vi "Modules Config.vi"(10 "Name":string, 11 "Module In":T1={"Names"={"Module Name"="", "Set Value"="", "Real Value"="", "FB Value"="", "Unit"="", "Identifier"="", "IdentifierW"="", "Decimal"="位数", "AS"=FALSE, "AR"=FALSE, "Con"=FALSE}, "Data"=[], "Digit"=0.0}) -> (2 "OK？":bool, 3 "Module Out":T1={"Names"={"Module Name"="", "Set Value"="", "Real Value"="", "FB Value"="", "Unit"="", "Identifier"="", "IdentifierW"="", "Decimal"="位数", "AS"=FALSE, "AR"=FALSE, "Con"=FALSE}, "Data"=[], "Digit"=0.0})   [LabVIEW 2020]
uses:
  0007 Controls/Data Modules.ctl
  0007 Controls/Data Element Single.ctl
  Global/Data Global/SDQ Data Type.ctl
panel:
  in  "InputBox":dbl
  in  "OK":bool
  in  "Cancel":bool
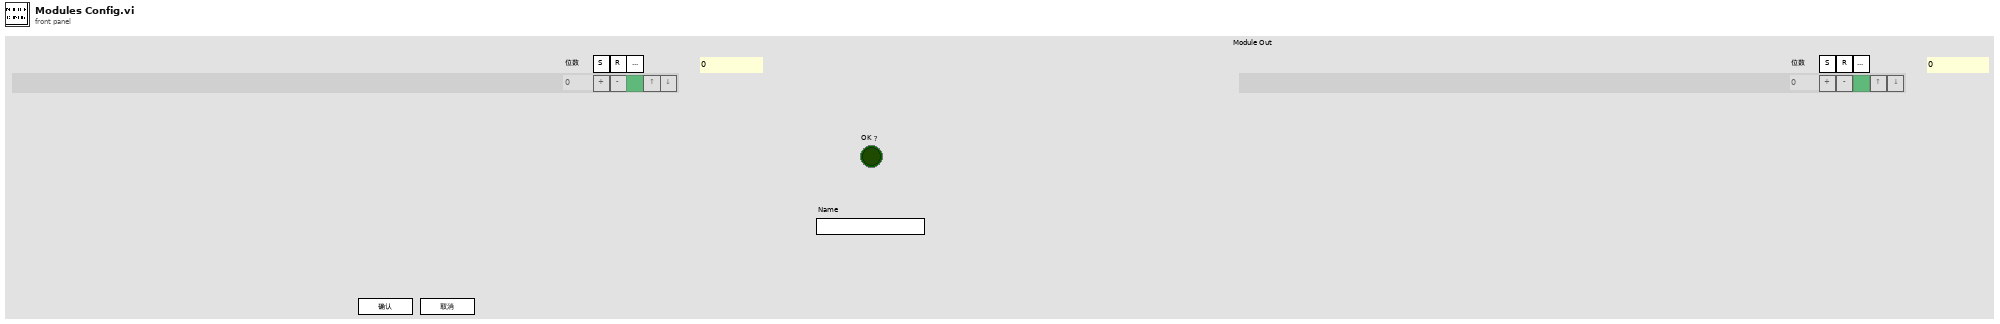
[diagram p1: front panel]
types:
  T1 = typedef "Data Modules.ctl" = cluster{"Names":cluster{"Module Name":string, "Set Value":string, "Real Value":string, "FB Value":string, "Unit":string, "Identifier":string, "IdentifierW":string, "Decimal":string, "AS":bool, "AR":bool, "Con":bool}, "Data":T2[], "Digit":dbl}
  T2 = typedef "Data Element Single.ctl" = cluster{"Name":string, "Set Value":string, "Real Value":string, "FB Value":string, "Unit":string, "Identifier":string, "Write Name":string, "Decimal":u16, "AS":bool, "AR":bool, "ALM":bool, "Up":bool, "Down":bool}
  T3 = typedef "SDQ Data Type.ctl" = cluster{"CAN Length":string, "CAN Name":string, "CAN ID":string, "CAN Type":string, "Test Item":string, "Byte Order":string, "Instruction":string, "Control Type":string, "Group":string, "Offset":dbl, "Coefficient":dbl, "Write Enable":bool, "Lable Type":string, "Key?":string, "Set Value":string, "Upper":dbl, "Lower":dbl, "Unit":string, "Formula":string, "Test Item Type":string, "Length":i32, "Address":string, "Name":string, "Identifier":string, "Data Type":string, "Enumerate?":string, "Enumerate List":string, "Data":string, "Source":string}
  T4 = cluster{"Active Row":i32, "Module In":T1, "TimeOut":i32, "List Visible":bool, "OK?":bool, "Active Column":i32, "Receive Data":map{string, T3}, "Data":refnum<vi>, "Name":string}
  T5 = enum8{"Enabled", "Disabled", "Disabled and Grayed Out"}
  T6 = enum32{"Invalid", "Default", "Floating", "Floating/Auto-Hide", "Modal"}
  T7 = cluster{"Name":bool, "Set Value":bool, "Real Value":bool, "FB Value":bool, "Unit":bool, "Identifier":bool, "Write Name":bool, "Decimal":bool, "AS":bool, "AR":bool, "ALM":bool, "Up":bool, "Down":bool}[]
  T8 = typedef "LVPoint32TypeDef.ctl" = cluster{"Horizontal":i32, "Vertical":i32}
  T9 = typedef "LVPositionTypeDef.ctl" = cluster{"Left":i32, "Top":i32}
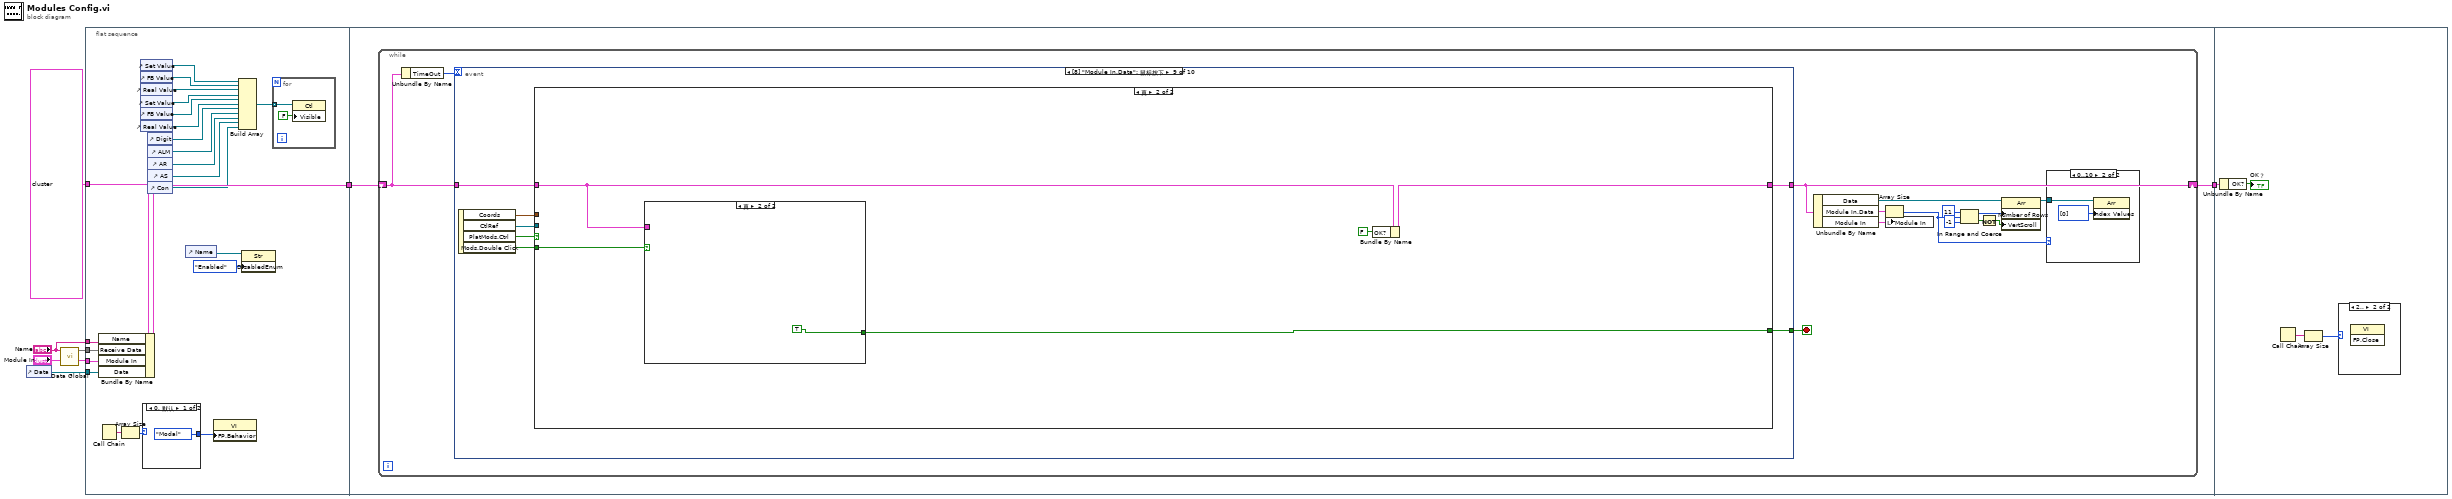
[diagram p0: block diagram]
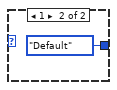
[diagram p2: hidden frame]
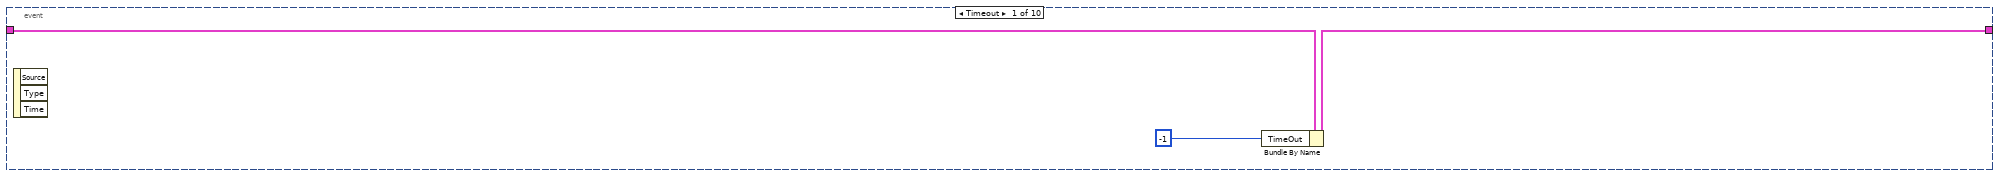
[diagram p3: hidden frame]
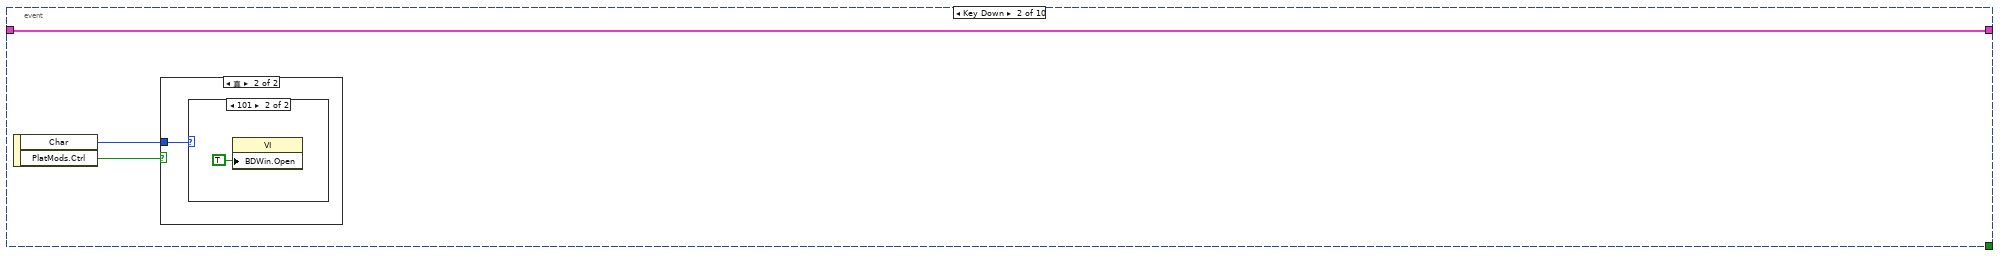
[diagram p4: hidden frame]
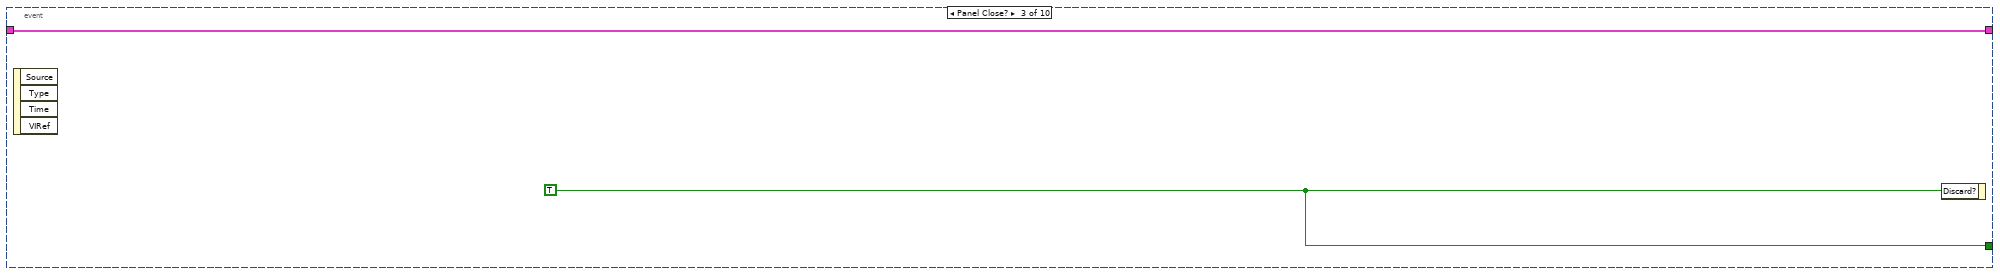
[diagram p7: hidden frame]
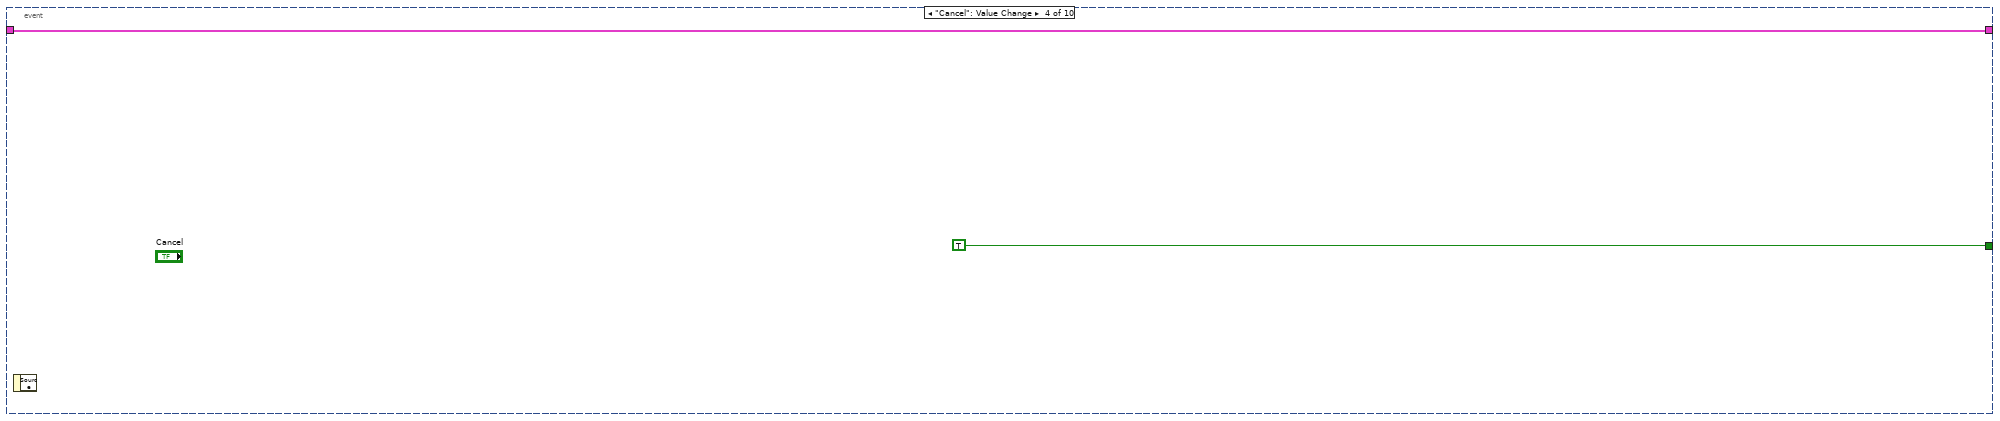
[diagram p8: hidden frame]
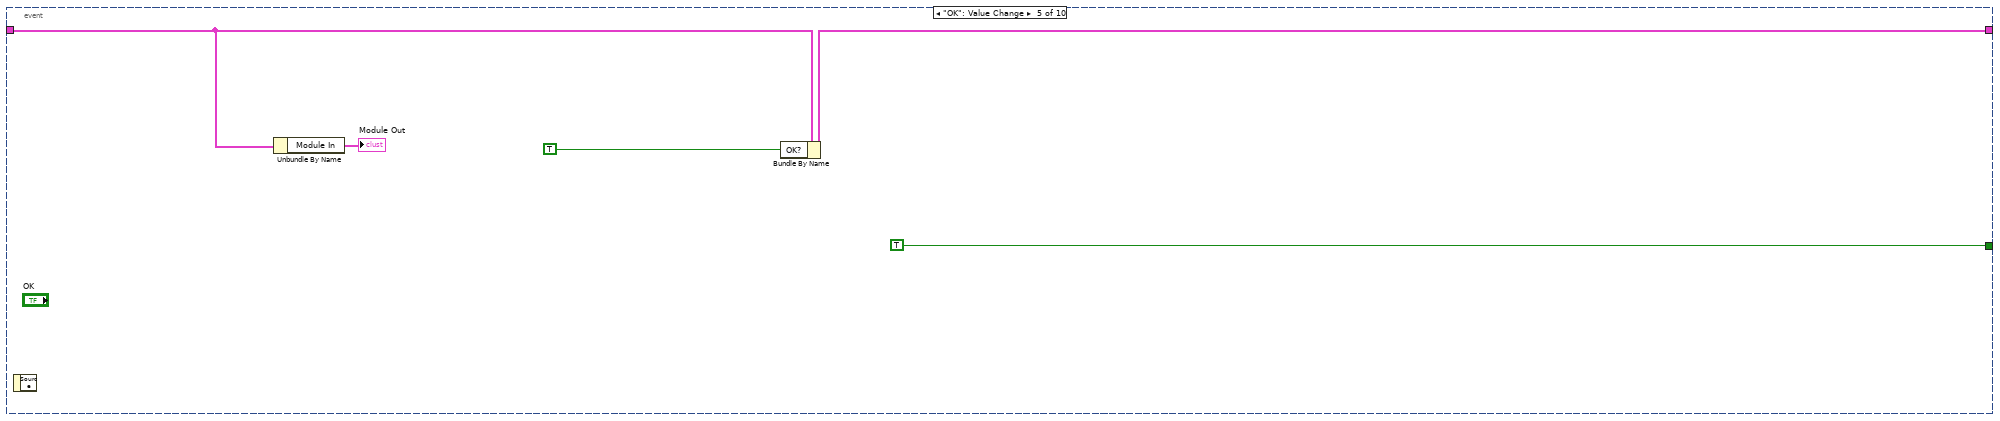
[diagram p9: hidden frame]
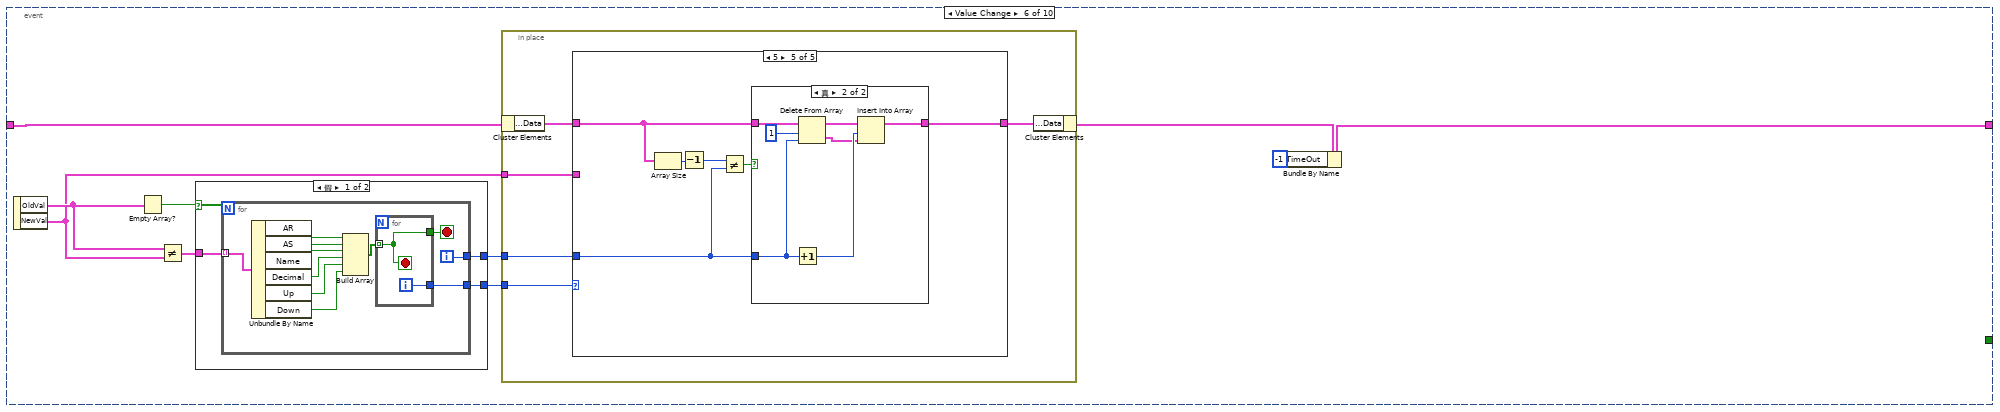
[diagram p10: hidden frame]
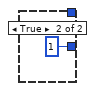
[diagram p11: hidden frame]
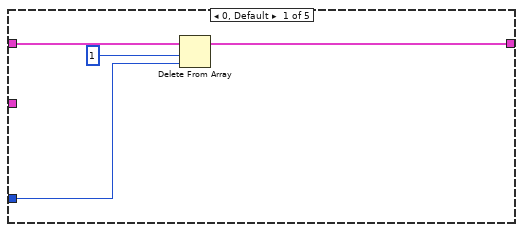
[diagram p12: hidden frame]
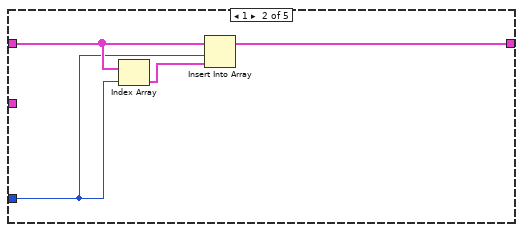
[diagram p13: hidden frame]
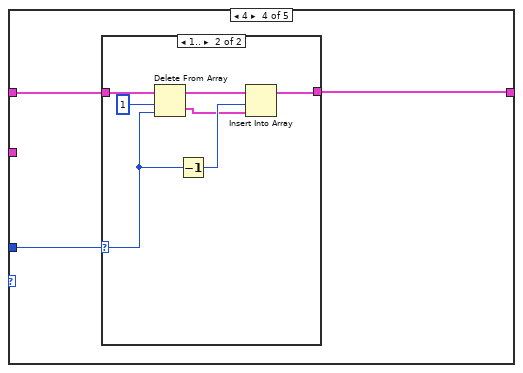
[diagram p15: hidden frame]
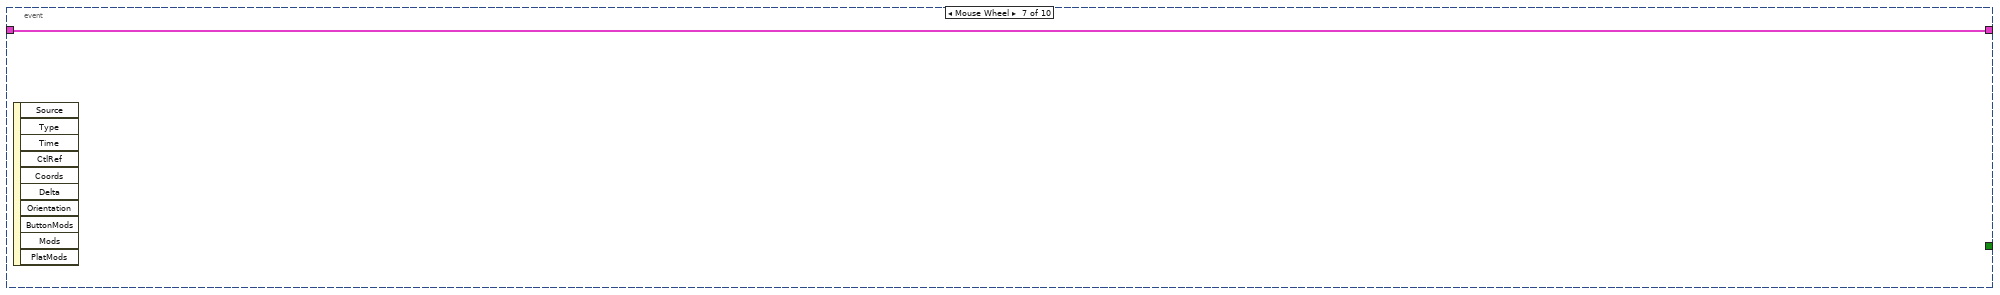
[diagram p18: hidden frame]
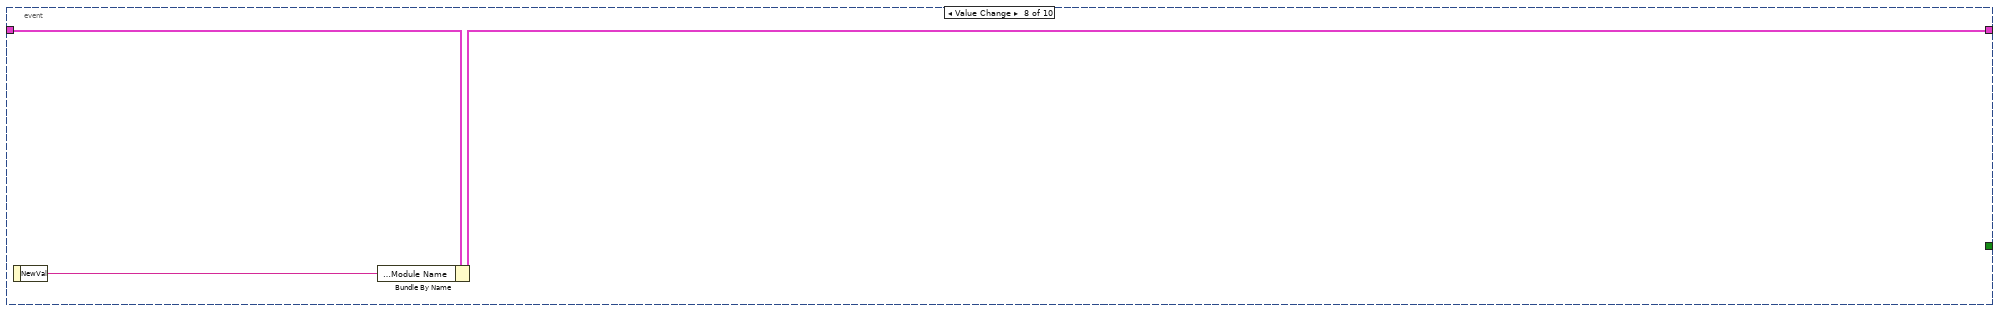
[diagram p19: hidden frame]
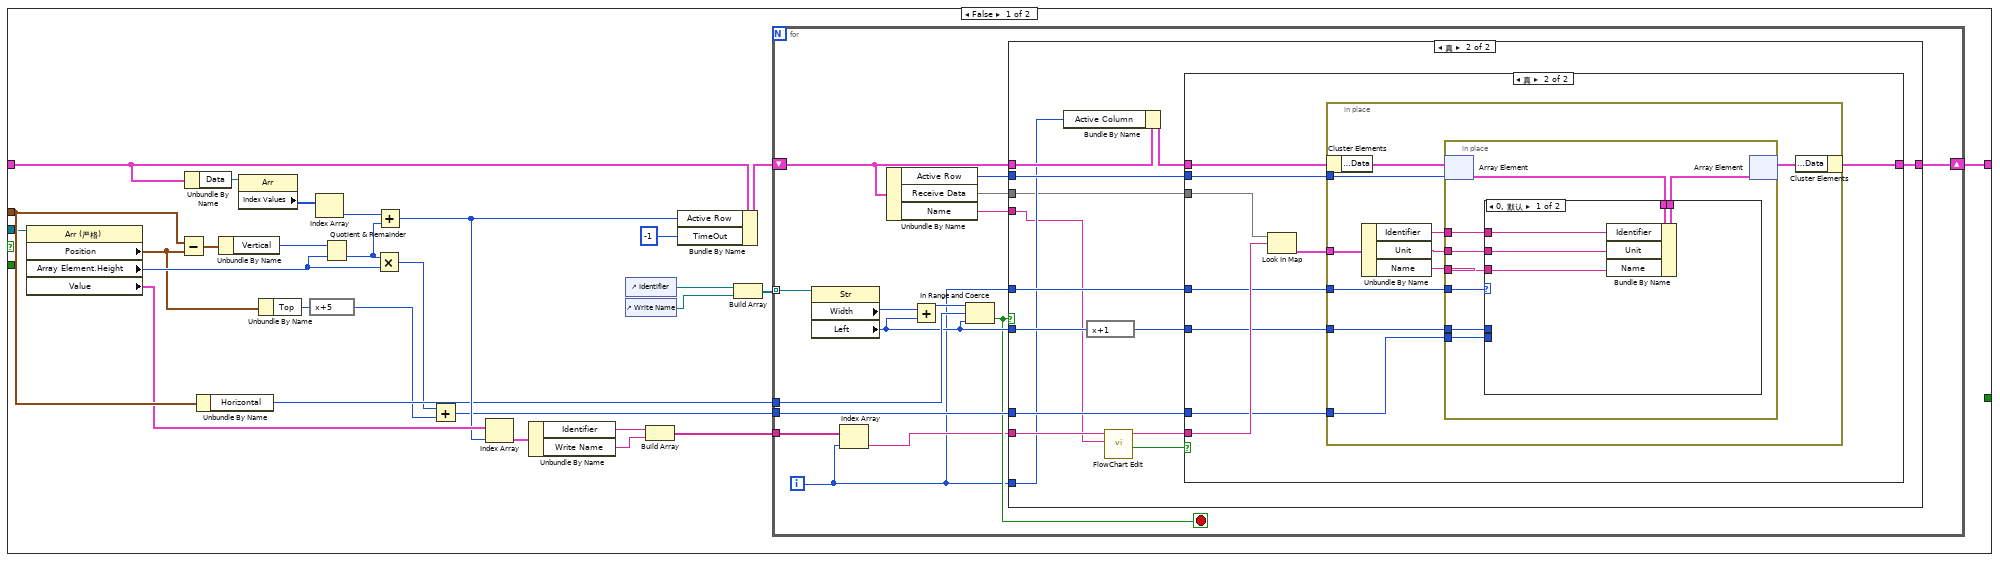
[diagram p20: hidden frame]
diagram:
  n1 = control-ref of="Data"() -> (w3:refnum<vi>)
  n2 = call "Data Global.vi"("Name"="Name") -> ("Data Out"=w2:map{string, T3})  [unwired: 7 in, 3 out]
  n3 = flat-sequence {
    tunnel: "Module In" -> [w28]
    tunnel: T4 {"Active Row"=0, "Module In"={"Names"={"Module Name"="", "Set Value"="", "Real Value"="", "FB Value"="", "Unit"="", "Identifier"="", "IdentifierW"="", "Decimal"="位数", "AS"=FALSE, "AR"=FALSE, "Con"=FALSE}, "Data"=[], "Digit"=0.0}, "TimeOut"=50, "List Visible"=FALSE, "OK?"=FALSE, "Active Column"=50, "Receive Data"={}, "Data"=refnum, "Name"=""} -> [w30]
    tunnel: [w29] -> w5
    tunnel: w2 -> [w25]
    tunnel: w3 -> [w24]
    tunnel: "Name" -> [w14]
    tunnel: w5 -> [w36]
    tunnel: [w35] -> w4
    tunnel: w4 -> [w266]
    frame #0 {
      n4 = Bundle By Name(cluster=w30, "Name"=w14, "Receive Data"=w25, "Module In"=w28, "Data"=w24) -> (w29:T4)
      n5 = Call Chain() -> (call chain=w27:string[])
      n6 = Array Size(array=w27) -> (size(s)=w26:i32)
      n7 = control-ref of="Set Value"() -> (w16:refnum<vi>)
      n8 = control-ref of="FB Value"() -> (w17:refnum<vi>)
      n9 = control-ref of="Real Value"() -> (w18:refnum<vi>)
      n10 = control-ref of="Set Value"() -> (w19:refnum<vi>)
      n11 = control-ref of="FB Value"() -> (w20:refnum<vi>)
      n12 = control-ref of="Real Value"() -> (w21:refnum<vi>)
      n13 = case shown="0, 默认" w26 {
        tunnel: [T6."Modal" ("前面板窗口:动作") T6."Default" ("前面板窗口:动作")] -> w15
        frame 0, Default {
        }
        frame 1 {
        }
      }
      n14 = control-ref of="AR"() -> (w12:refnum<vi>)
      n15 = control-ref of="Con"() -> (w10:refnum<vi>)
      n16 = control-ref of="Digit"() -> (w22:refnum<vi>)
      n17 = control-ref of="ALM"() -> (w13:refnum<vi>)
      n18 = control-ref of="AS"() -> (w11:refnum<vi>)
      n19 = control-ref of="Name"() -> (w9:refnum<vi>)
      n20 = property class="VI"("FP.Behavior"=w15) -> ()  [unwired: 2 in, 2 out]
      n21 = Build Array(w16, w17, w18, w19, w20, w21, w22, w13, w12, w11, w10) -> (w23:refnum<vi>[])
      n22 = property class="Str"(reference=w9, "DisabledEnum"=T5."Enabled" ("禁用")) -> ()  [unwired: 1 in, 2 out]
      n23 = for {
        tunnel: w23 -> [w32] mode=indexing
        n24 = property class="Ctl"(reference=w32, "Visible"=FALSE ("可见")) -> ()  [unwired: 1 in, 2 out]
      }
    }
    frame #1 {
      n25 = while {
        shift-right: [w49] -> w35
        shift-left: w36 -> [w48]
        stop <- w50 stop-if-true
        n26 = Unbundle By Name(w48) -> ("TimeOut"=w47:i32)
        n27 = event shown="[8] \"Module In.Data\": 鼠标按下" {
          selector: _ -> [_ _ _ _ _ _ _ _ _ _]
          dyn-events: _ -> [_ _ _ _ _ _ _ _ _ _]
          timeout: w47 -> [_ _ _ _ _ _ _ _ _ _]
          tunnel: [_ _ w60 TRUE ("放弃？") TRUE ("放弃？") _ _ _ w138 _] -> w50
          tunnel: w48 -> [w53 w56 w59 w61 w66 w74 w134 w137 w141 w248]
          tunnel: [w52 w56 w59 w61 w64 w76 w134 w136 w142 w249] -> w49
          event Timeout {
            n28 = event-data() -> ()  [unwired: 1 in, 3 out]
            n29 = Bundle By Name(cluster=w53, "TimeOut"=-1) -> (w52:T4)
          }
          event Key Down {
            n30 = event-data() -> ("Char"=w55:i16, "PlatMods.Ctrl"=w54:bool)  [unwired: 1 in]
            n31 = case shown="真" w54 {
              tunnel: w55 -> [_ w57]
              frame False {
              }
              frame True {
                n32 = case shown="101" w57 {
                  frame 0, Default {
                  }
                  frame 101 {
                    n33 = property class="VI"("BDWin.Open"=TRUE ("程序框图窗口:打开")) -> ()  [unwired: 2 in, 2 out]
                  }
                }
              }
            }
          }
          event Panel Close? {
            w60 = TRUE ("放弃？")
            n34 = event-data() -> ()  [unwired: 1 in, 4 out]
            n35 = event-data("Discard?"=w60) -> ()  [unwired: 1 in, 1 out]
          }
          event "Cancel": Value Change {
            n36 = event-data() -> ()  [unwired: 1 in, 1 out]
          }
          event "OK": Value Change {
            n37 = event-data() -> ()  [unwired: 1 in, 1 out]
            n38 = Unbundle By Name(w66) -> ("Module In"=→"Module Out":T1)
            n39 = Bundle By Name(cluster=w66, "OK?"=TRUE) -> (w64:T4)
          }
          event Value Change {
            n40 = event-data() -> ("OldVal"=w73:T2[], "NewVal"=w71:T2[])  [unwired: 1 in]
            n41 = Empty Array?(array=w73) -> (empty?=w70:bool)
            n42 = Not Equal?(x=w73, y=w71) -> (x != y?=w72:T7)
            n43 = case shown="假" w70 {
              tunnel: [w80 _] -> w69
              tunnel: w72 -> [w79 _]
              tunnel: [w78 1] -> w68
              frame False {
                n44 = for {
                  tunnel: [w91] -> w80
                  tunnel: w79 -> [w90] mode=indexing
                  tunnel: [w84] -> w78
                  i -> [w91]
                  stop <- w85 stop-if-true
                  n45 = Unbundle By Name(w90) -> ("AR"=w89:bool, "AS"=w88:bool, "Name"=w87:bool, "Decimal"=w83:bool, "Up"=w82:bool, "Down"=w81:bool)
                  n46 = Build Array(w89, w88, w87, w83, w82, w81) -> (w86:bool[])
                  n47 = for {
                    tunnel: w86 -> [w93] mode=indexing
                    tunnel: [w93] -> w85
                    tunnel: [w92] -> w84
                    i -> [w92]
                    stop <- w93 stop-if-true
                  }
                }
              }
              frame True {
              }
            }
            n48 = in-place {
              in-place-border: w69 -> [w97]
              in-place-border: w68 -> [w96]
              in-place-border: w71 -> [w95]
              n49 = in-place-cluster #1(w74) -> ("Module In.Data"=w99:T2[])
              n50 = case shown="5" w96 {
                tunnel: w99 -> [w103 w106 _ w110 w122]
                tunnel: [w102 w107 w108 w109 w121] -> w98
                tunnel: w97 -> [w101 w104 _ w111 w120]
                tunnel: w95 -> [_ _ w108 _ _]
                frame 0, Default {
                  n51 = Delete From Array(array=w103, length=1 ("长度"), index=w101) -> (array with subset deleted=w102:T2[])  [unwired: 1 out]
                }
                frame 1 {
                  n52 = Index Array(array=w106, index=w104) -> (element=w105:T2)
                  n53 = Insert Into Array(array=w106, index=w104, new element=w105) -> (w107:T2[])
                }
                frame 2, 3 {
                }
                frame 4 {
                  n54 = case shown="1.." w111 {
                    selector: w111 -> [_ w114]
                    tunnel: [w112 w116] -> w109
                    tunnel: w110 -> [w112 w119]
                    frame 0, Default {
                    }
                    frame 1.. {
                      n55 = Delete From Array(array=w119, length=1 ("长度"), index=w114) -> (deleted portion=w115:T2[], array with subset deleted=w118:T2[])
                      n56 = Decrement(x=w114) -> (x-1=w117:i32)
                      n57 = Insert Into Array(array=w118, index=w117, new element=w115) -> (w116:T2[])
                    }
                  }
                }
                frame 5 {
                  n58 = Array Size(array=w122) -> (size(s)=w125:i32)
                  n59 = Decrement(x=w125) -> (x-1=w124:i32)
                  n60 = Not Equal?(x=w124, y=w120) -> (x != y?=w123:bool)
                  n61 = case shown="真" w123 {
                    tunnel: w122 -> [w126 w133]
                    tunnel: [w126 w127] -> w121
                    tunnel: w120 -> [_ w130]
                    frame False {
                    }
                    frame True {
                      n62 = Increment(x=w130) -> (x+1=w129:i32)
                      n63 = Delete From Array(array=w133, length=1 ("长度"), index=w130) -> (deleted portion=w128:T2[], array with subset deleted=w132:T2[])
                      n64 = Insert Into Array(array=w132, index=w129, new element=w128) -> (w127:T2[])
                    }
                  }
                }
              }
              n65 = in-place-cluster #1("Module In.Data"=w98) -> (w77:T4)
            }
            n66 = Bundle By Name(cluster=w77, "TimeOut"=-1) -> (w76:T4)
          }
          event Mouse Wheel {
            n67 = event-data() -> ()  [unwired: 1 in, 10 out]
          }
          event Value Change {
            n68 = event-data() -> ("NewVal"=w135:string)  [unwired: 1 in]
            n69 = Bundle By Name(cluster=w137, "Module In.Names.Module Name"=w135) -> (w136:T4)
          }
          event Mouse Down {
            n70 = event-data() -> ("Coords"=w144:T8, "CtlRef"=w143:refnum<vi>, "PlatMods.Ctrl"=w140:bool, "Mods.Double Click"=w139:bool)  [unwired: 1 in]
            n71 = case shown="真" w140 {
              tunnel: w144 -> [w172 _]
              tunnel: w143 -> [w171 _]
              tunnel: [w170 w241] -> w142
              tunnel: w141 -> [w148 w239]
              tunnel: w139 -> [_ w243]
              tunnel: [_ w242] -> w138
              frame False {
                n72 = property class="Arr (严格)"(reference=w171) -> ("Position"=w150:T9, "Array Element.Height"=w154:u32, "Value"=w163:T2[])  [unwired: 1 in, 2 out]
                n73 = Subtract(x=w172, y=w150) -> (x-y=w169:T8)
                n74 = Unbundle By Name(w148) -> ("Data"=w147:refnum<vi>)
                n75 = Unbundle By Name(w172) -> ("Horizontal"=w156:i32)
                n76 = Unbundle By Name(w169) -> ("Vertical"=w168:i32)
                n77 = property on="属性节点" class="Arr"(reference=w147) -> ("Index Values"=w165:u32[])  [unwired: 1 in, 2 out]
                n78 = Unbundle By Name(w150) -> ("Top"=w152:i32)
                n79 = expression code="x+5"(w152) -> (w149:i32)
                n80 = Index Array(array=w165) -> (element=w164:u32)  [unwired: 1 in]
                n81 = Quotient & Remainder(x=w168, y=w154) -> (floor(x/y)=w155:u32)  [unwired: 1 out]
                n82 = Multiply(x=w155, y=w154) -> (x*y=w153:u32)
                n83 = Add(x=w164, y=w155) -> (x+y=w162:u32)
                n84 = Add(x=w153, y=w149) -> (x+y=w151:u32)
                n85 = Index Array(array=w163, index=w162) -> (element=w167:T2)
                n86 = Unbundle By Name(w167) -> ("Identifier"=w161:string, "Write Name"=w160:string)
                n87 = control-ref of="Identifier"() -> (w146:refnum<vi>)
                n88 = control-ref of="Write Name"() -> (w145:refnum<vi>)
                n89 = Build Array(w161, w160) -> (w159:string[])
                n90 = Bundle By Name(cluster=w148, "Active Row"=w162, "TimeOut"=-1) -> (w157:T4)
                n91 = Build Array(w146, w145) -> (w158:refnum<vi>[])
                n92 = for {
                  tunnel: w159 -> [w176]
                  tunnel: w158 -> [w185] mode=indexing
                  tunnel: w156 -> [w184]
                  shift-right: [w183] -> w170
                  shift-left: w157 -> [w182]
                  tunnel: w151 -> [w178]
                  i -> [w174]
                  stop <- w177 stop-if-true
                  n93 = property class="Str"(reference=w185) -> ("Width"=w187:u32, "Left"=w179:i32)  [unwired: 1 in, 2 out]
                  n94 = Index Array(array=w176, index=w174) -> (element=w175:string)
                  n95 = Unbundle By Name(w182) -> ("Active Row"=w180:i32, "Receive Data"=w181:map{string, T3}, "Name"=w173:string)
                  n96 = Add(x=w187, y=w179) -> (x+y=w186:u32)
                  n97 = In Range and Coerce(upper limit=w186, x=w184, lower limit=w179) -> (In Range?=w177:bool)  [unwired: 1 out]
                  n98 = case shown="真" w177 {
                    tunnel: w175 -> [_ w202]
                    tunnel: w182 -> [w188 w201]
                    tunnel: [w188 w200] -> w183
                    tunnel: w181 -> [_ w190]
                    tunnel: w180 -> [_ w197]
                    tunnel: w174 -> [_ w196]
                    tunnel: w179 -> [_ w195]
                    tunnel: w178 -> [_ w194]
                    tunnel: w174 -> [_ w191]
                    tunnel: w173 -> [_ w189]
                    frame False {
                    }
                    frame True {
                      n99 = Bundle By Name(cluster=w201, "Active Column"=w191) -> (w192:T4)
                      n100 = expression code="x+1"(w195) -> (w193:i32)
                      n101 = call "FlowChart Edit.vi"("Name"=w189, "Identifier In"=w202) -> ("OK？"=w199:bool, "Identifier Out"=w198:string)  [unwired: 6 in, 2 out]
                      n102 = case shown="真" w199 {
                        tunnel: w192 -> [w203 w212]
                        tunnel: [w203 w211] -> w200
                        tunnel: w198 -> [_ w209]
                        tunnel: w190 -> [_ w210]
                        tunnel: w197 -> [_ w208]
                        tunnel: w196 -> [_ w206]
                        tunnel: w193 -> [_ w205]
                        tunnel: w194 -> [_ w204]
                        frame False {
                        }
                        frame True {
                          n103 = Look In Map(map=w210, key=w209) -> (value=w207:T3)  [unwired: 1 in, 1 out]
                          n104 = in-place {
                            in-place-border: w208 -> [w220]
                            in-place-border: w207 -> [w219]
                            in-place-border: w206 -> [w215]
                            in-place-border: w205 -> [w214]
                            in-place-border: w204 -> [w213]
                            n105 = in-place-cluster #2(w212) -> ("Module In.Data"=w222:T2[])
                            n106 = Unbundle By Name(w219) -> ("Identifier"=w218:string, "Unit"=w217:string, "Name"=w216:string)
                            n107 = in-place {
                              in-place-border: w218 -> [w228]
                              in-place-border: w217 -> [w227]
                              in-place-border: w216 -> [w226]
                              in-place-border: w215 -> [w225]
                              in-place-border: w214 -> [w224]
                              in-place-border: w213 -> [w223]
                              n108 = in-place-array #3(w222, w220) -> (w230:T2)
                              n109 = case shown="0, 默认" w225 {
                                tunnel: w230 -> [w235 w238]
                                tunnel: [w234 w237] -> w229
                                tunnel: w228 -> [w233 w236]
                                tunnel: w227 -> [w232 _]
                                tunnel: w226 -> [w231 _]
                                tunnel: w224 -> [_ _]
                                tunnel: w223 -> [_ _]
                                frame 0, Default {
                                n110 = Bundle By Name(cluster=w235, "Identifier"=w233, "Unit"=w232, "Name"=w231) -> (w234:T2)
                                }
                                frame 1 {
                                n111 = Bundle By Name(cluster=w238, "Write Name"=w236) -> (w237:T2)
                                }
                              }
                              n112 = in-place-array #3(w229) -> (w221:T2[])  [unwired: 1 out]
                            }
                            n113 = in-place-cluster #2("Module In.Data"=w221) -> (w211:T4)
                          }
                        }
                      }
                    }
                  }
                }
              }
              frame True {
                n114 = case shown="真" w243 {
                  tunnel: [_ TRUE] -> w242
                  tunnel: w239 -> [_ _]
                  frame False {
                  }
                  frame True {
                  }
                }
                n115 = Bundle By Name(cluster=w239, "OK?"=FALSE) -> (w241:T4)
              }
            }
          }
          event "InputBox": Value Change {
            n116 = event-data() -> ()  [unwired: 1 in, 1 out]
            n117 = Format Into String(format string="%#.6f" ("格式字符串"), "InputBox") -> (resulting string=w245:string)  [unwired: 2 in, 1 out]
            n118 = in-place {
              in-place-border: w248 -> [w254]
              in-place-border: w245 -> [w250]
              n119 = in-place-cluster #4(w248) -> ("Module In.Data"=w255:T2[])
              n120 = Unbundle By Name(w254) -> ("Active Row"=w253:i32, "Active Column"=w251:i32)
              n121 = in-place {
                in-place-border: w251 -> [w257]
                in-place-border: w250 -> [w256]
                n122 = in-place-array #5(w255, w253) -> (w259:T2)
                n123 = case shown="0, 默认" w257 {
                  tunnel: w259 -> [w260]
                  tunnel: [w260] -> w258
                  tunnel: w256 -> [_]
                  frame 0, Default {
                  }
                }
                n124 = in-place-array #5(w258) -> (w252:T2[])  [unwired: 1 out]
              }
              n125 = in-place-cluster #4("Module In.Data"=w252) -> (w249:T4)
            }
          }
        }
        n126 = Unbundle By Name(w49) -> ("Data"=w39:refnum<vi>, "Module In.Data"=w46:T2[], "Module In"=w37:T1)
        n127 = Array Size(array=w46) -> (size(s)=w40:i32)
        n128 = local write "Module In"(w37) -> ()
        n129 = In Range and Coerce(upper limit=11 ("行数"), x=w40, lower limit=-1 ("行数")) -> (coerced(x)=w41:i32, In Range?=w43:bool)
        n130 = Not(x=w43) -> (.not. x?=w42:bool)
        n131 = property on="属性节点" class="Arr"(reference=w39, "Number of Rows"=w41, "VertScroll"=w42) -> (reference out=w38:refnum<vi>)  [unwired: 1 in, 1 out]
        n132 = case shown="0..10" w40 {
          tunnel: w38 -> [_ w261]
          frame 999, Default {
          }
          frame 0..10 {
            n133 = property on="属性节点" class="Arr"(reference=w261, "Index Values"=u32[] [0] ("索引值")) -> ()  [unwired: 1 in, 2 out]
          }
        }
      }
    }
    frame #2 {
      n134 = Unbundle By Name(w266) -> ("OK?"=→"OK？":bool)
      n135 = Call Chain() -> (call chain=w264:string[])
      n136 = Array Size(array=w264) -> (size(s)=w263:i32)
      n137 = case shown="2.." w263 {
        frame 0, Default {
        }
        frame 2.. {
          n138 = invoke class="VI" method="FP.Close"() -> ()  [unwired: 3 in, 3 out]
        }
      }
    }
  }
